vi "强度图的使用.vi"() -> ()   [LabVIEW 2018]
panel:
  in  "停止":bool
  out "强度图":dbl[][](graph)
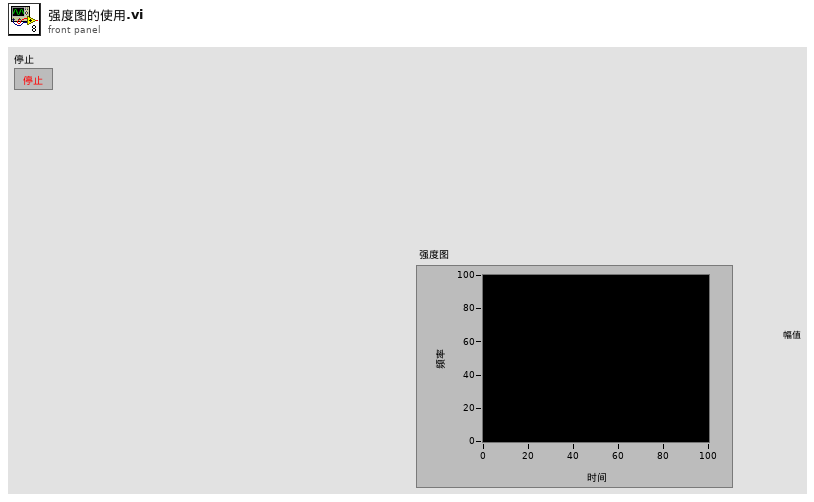
[diagram p1: front panel]
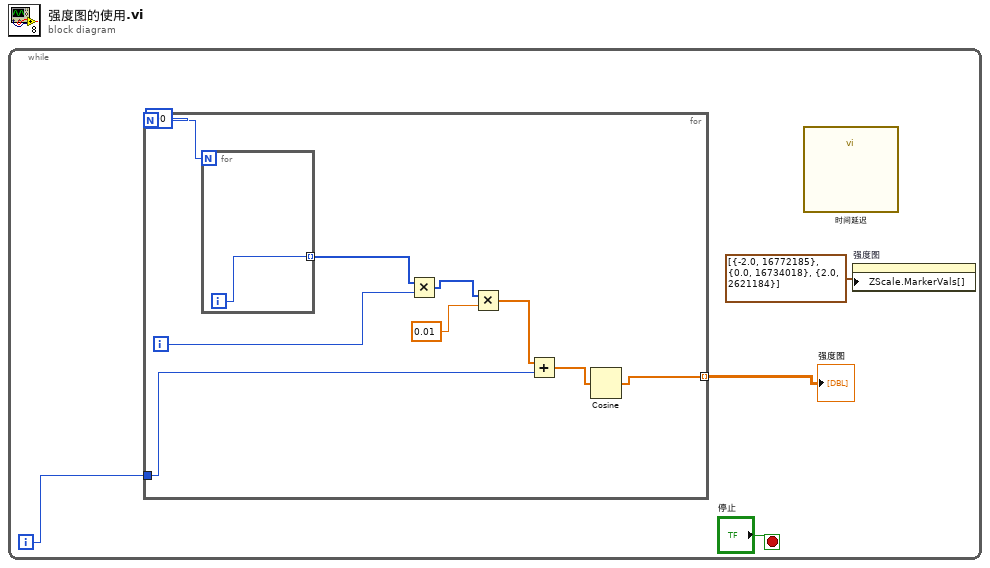
[diagram p0: block diagram]
diagram:
  n1 = while {
    i -> [w3]
    stop <- "停止" stop-if-true
    n2 = for {
      N: 100 -> [w14]
      tunnel: w3 -> [w9]
      tunnel: [w6] -> w2 mode=indexing
      i -> [w12]
      n3 = for {
        N: w14 -> [_]
        tunnel: [w15] -> w13 mode=indexing
        i -> [w15]
      }
      n4 = Multiply(x=w13, y=w12) -> (x*y=w10:i32[])
      n5 = Multiply(x=w10, y=0.01) -> (x*y=w8:dbl[])
      n6 = Add(x=w8, y=w9) -> (x+y=w7:dbl[])
      n7 = Cosine(x=w7) -> (cos(x)=w6:dbl[])
    }
    "强度图" <- w2
    n8 = call "时间延迟"() -> ()  [unwired: 11 in, 1 out]
    n9 = property on="强度图" class="IntGraph (严格)"("ZScale.MarkerVals[]"=cluster{dbl, u32}[] [{-2.0, 16772185}, {0.0, 16734018}, {2.0, 2621184}] ("Z标尺.刻度值[]")) -> ()  [unwired: 2 in, 2 out]
  }
